vi "OutputError.vi"(8 "error in (no error)":errorcluster, 9 "Causing VI":string, 10 "Calling VI":string) -> (0 "error out":errorcluster)   [LabVIEW 2015]
doc: "Sends any errors that occur to the SmartDashboard. If the error, calling VI, and causing VI is identical to a previous error, the error will not be sent."
uses:
  <vilib>/Rock Robotics/Network Tables/SD Write Numeric Array.vi
  <vilib>/Rock Robotics/Network Tables/SD Write Boolean Array.vi
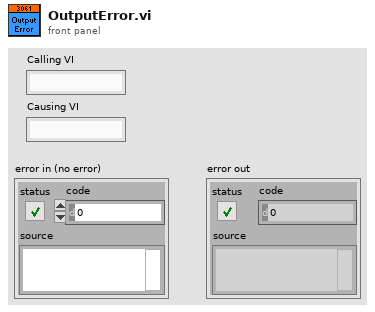
[diagram p1: front panel]
types:
  T1 = cluster{"Boolean":bool, "Numeric":i32, "String":string}
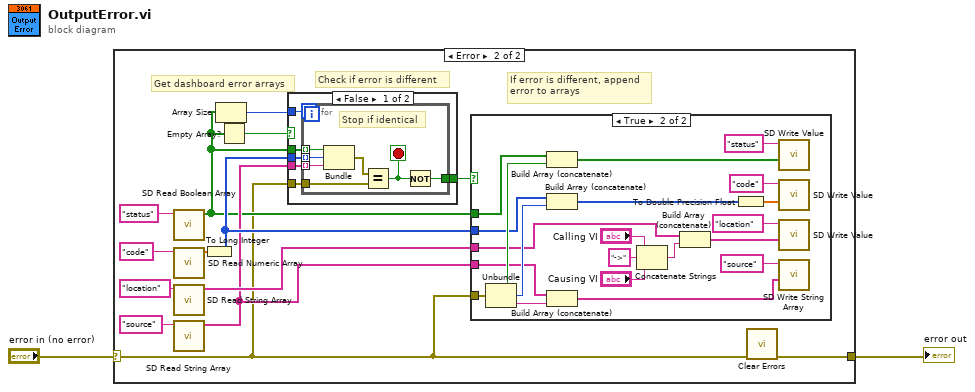
[diagram p0: block diagram]
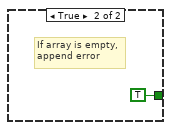
[diagram p3: hidden frame]
diagram:
  n1 = case shown="Error" "error in (no error)" {
    selector: "error in (no error)" -> [w3 w4]
    tunnel: [w3 w5] -> w2
    frame No Error {
    }
    frame Error {
      # "Check if error is different"
      # "If error is different, append\nerror to arrays"
      # "Get dashboard error arrays"
      n2 = call <vilib>:"SD Read Boolean Array.vi"("Name"="status") -> ("Boolean Array"=w7:bool[])  [unwired: 8 in, 2 out]
      n3 = call <vilib>:"SD Read Numeric Array.vi"("Name"="code") -> ("Numeric Array"=w14:dbl[])  [unwired: 8 in, 2 out]
      n4 = call <vilib>:"SD Read String Array.vi"("Name"="location") -> ("String Array"=w10:string[])  [unwired: 9 in, 1 out]
      n5 = call <vilib>:"SD Read String Array.vi"("Name"="source") -> ("String Array"=w9:string[])  [unwired: 9 in, 1 out]
      n6 = To Long Integer(number=w14) -> (32bit integer=w12:i32[])
      n7 = Array Size(array=w7) -> (size(s)=w8:i32)
      n8 = Empty Array?(array=w7) -> (empty?=w6:bool)
      n9 = case shown="False" w6 {
        tunnel: w8 -> [w23 _]
        tunnel: w4 -> [w22 _]
        tunnel: [w21 TRUE] -> w13
        tunnel: w7 -> [w20 _]
        tunnel: w12 -> [w19 _]
        tunnel: w9 -> [w18 _]
        frame False {
          n10 = for {
            N: w23 -> [_]
            tunnel: w22 -> [w27]
            tunnel: w20 -> [w30] mode=indexing
            tunnel: w19 -> [w29] mode=indexing
            tunnel: w18 -> [w28] mode=indexing
            tunnel: [w24] -> w21
            stop <- w25 stop-if-true
            # "Stop if identical"
            n11 = Bundle("Boolean"=w30, "Numeric"=w29, "String"=w28) -> (w26:T1)  [unwired: 1 in]
            n12 = Equal?(x=w26, y=w27) -> (x = y?=w25:bool)
            n13 = Not(x=w25) -> (.not. x?=w24:bool)
          }
        }
        frame True {
          # "If array is empty,\nappend error"
        }
      }
      n14 = case shown="True" w13 {
        tunnel: w4 -> [_ w52]
        tunnel: w7 -> [_ w45]
        tunnel: w12 -> [_ w42]
        tunnel: w10 -> [_ w35]
        tunnel: w9 -> [_ w36]
        frame False {
        }
        frame True {
          n15 = Unbundle(w52) -> ("status"=w44:bool, "code"=w41:i32, "source"=w37:string)
          n16 = Build Array (concatenate)(w45, w44) -> (w43:bool[])
          n17 = Build Array (concatenate)(w42, w41) -> (w40:i32[])
          n18 = Build Array (concatenate)(w36, w37) -> (w33:string[])
          n19 = Concatenate Strings("Calling VI", "->" ("string"), "Causing VI") -> (w34:string)
          n20 = Build Array (concatenate)(w35, w34) -> (w32:string[])
          n21 = To Double Precision Float(number=w40) -> (double precision float=w39:dbl[])
          n22 = call-poly <vilib>:"SD Write Value.vi"("Boolean Array"=w43, "Name"="status") -> ()  [unwired: 8 in, 2 out]
          n23 = call-poly <vilib>:"SD Write Value.vi"("Numeric Array"=w39, "Name"="code") -> ()  [unwired: 8 in, 2 out]
          n24 = call-poly <vilib>:"SD Write Value.vi"("String Array"=w32, "Name"="location") -> ()  [unwired: 8 in, 2 out]
          n25 = call <vilib>:"SD Write String Array.vi"("String Array"=w33, "Name"="source") -> ()  [unwired: 8 in, 2 out]
        }
      }
      n26 = call <vilib>:"Clear Errors.vi"("error in (no error)"=w4) -> ("error out"=w5:errorcluster)  [unwired: 5 in, 1 out]
    }
  }
  "error out" <- w2
